vi "LVFunction_Imop_SlopesCompute_ModalCoef.vi"(0 "HasoSlopes IN":refnum<class "HasoSlopes.lvclass">, 5 "ComputePhaseSet":refnum<class "ComputePhaseSet.lvclass">, 7 "ModalCoef  IN":refnum<class "ModalCoef.lvclass">, 11 "error constant":errorcluster) -> (4 "HasoSlopes (dup)":refnum<class "HasoSlopes.lvclass">, 6 "ComputePhaseSet.lvclass (dup)":refnum<class "ComputePhaseSet.lvclass">, 8 "ModalCoef OUT":refnum<class "ModalCoef.lvclass">, 15 "error out":errorcluster)   [LabVIEW 2020]
doc: "Compute modal coefficients that represent the processed slopes of the input\nslopes data in a given basis of polynomials provided by ComputePhaseSet.\n\n<B>ComputePhaseSetIn</B> : ComputePhaseSet object.\n<B>ComputePhaseSetOut</B> : ComputePhaseSet object.\n<B>HasoData</B> : Slopes object.\n<B>ModalCoeffs</B> : ModalCoef object. Preferences are used as input, coefficients values are updated by the processing."
uses:
  HasoSlopes.lvclass
  ComputePhaseSet.lvclass
  ModalCoef.lvclass
  LVClass_ModalCoef Read ModalCoef.vi
  LVClass_ComputePhaseSet Read ComputePhaseSet.vi
  LVClass_HasoSlopes Read HasoSlopes _ property.vi
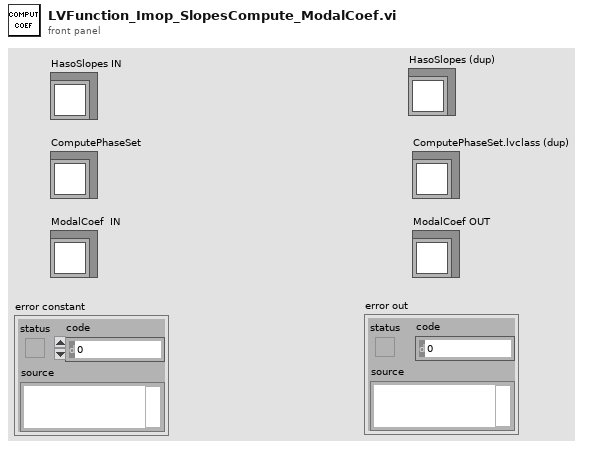
[diagram p1: front panel]
types:
  T1 = typedef "ClassID.ctl" = i64
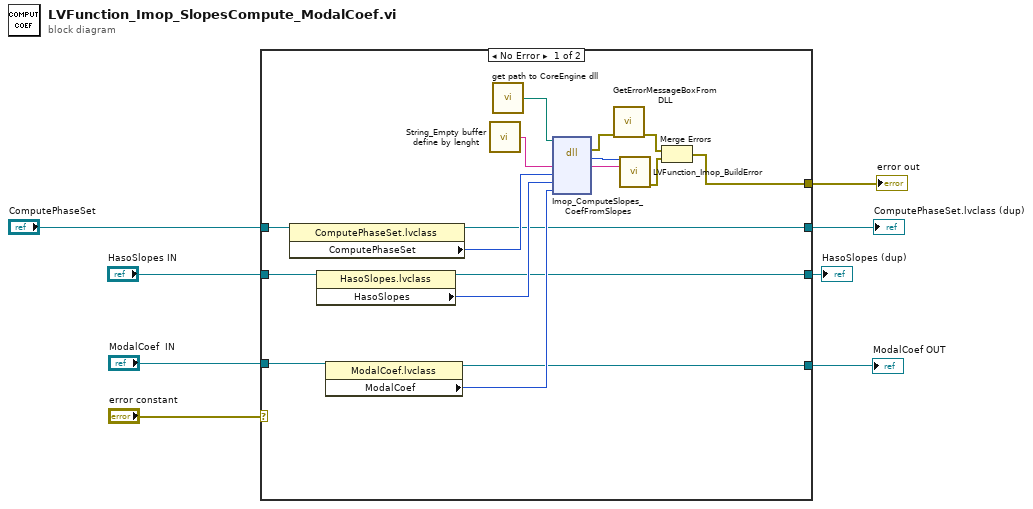
[diagram p0: block diagram]
diagram:
  n1 = case shown="No Error" "error constant" {
    selector: "error constant" -> [_ w29]
    tunnel: "HasoSlopes IN" -> [w20 w26]
    tunnel: "ComputePhaseSet" -> [w19 w28]
    tunnel: [w12 w29] -> w7
    tunnel: "ModalCoef  IN" -> [w16 w27]
    tunnel: [w11 w27] -> w3
    tunnel: [w10 w28] -> w2
    tunnel: [w9 w26] -> w1
    frame No Error {
      n2 = property class="ComputePhaseSet.lvclass"(reference=w19) -> (reference out=w10:refnum<class "ComputePhaseSet.lvclass">, "ComputePhaseSet"=w18:T1)  [unwired: 1 in, 1 out]
      n3 = property class="HasoSlopes.lvclass"(reference=w20) -> (reference out=w9:refnum<class "HasoSlopes.lvclass">, "HasoSlopes"=w17:T1)  [unwired: 1 in, 1 out]
      n4 = property class="ModalCoef.lvclass"(reference=w16) -> (reference out=w11:refnum<class "ModalCoef.lvclass">, "ModalCoef"=w15:T1)  [unwired: 1 in, 1 out]
      n5 = call "String_Empty buffer define by lenght.vi"() -> ("Empty buffer"=w23:string)  [unwired: 1 in]
      n6 = call "get path to CoreEngine dll.vi"() -> ("path to wavekit library"=w22:path)  [unwired: 14 in, 1 out]
      n7 = dll-call lib="D:/FLE/0.Code/CoreEngine4_Suite/LV2011_interface/DLLs/c_interface_vc100.dll" fn="Imop_ComputeSlopes_CoefFromSlopes"(path in=w22, "message"=w23, "ComputePhaseSet"=w18, "HasoSlopes"=w17, "ModalCoeffs"=w15) -> (error out=w21:errorcluster, "return type"=w25:i32, "message"=w24:string)  [unwired: 5 in, 1 out]
      n8 = call "GetErrorMessageBoxFromDLL.vi"("error IN"=w21) -> ("error OUT"=w14:errorcluster)  [unwired: 10 in]
      n9 = call "LVFunction_Imop_BuildError.vi"("code"=w25, "String to Prepend to source (\"\")"=w24) -> ("error out"=w13:errorcluster)  [unwired: 13 in]
      n10 = Merge Errors(w14, w13) -> (w12:errorcluster)
    }
    frame Error {
    }
  }
  "error out" <- w7
  "ModalCoef OUT" <- w3
  "ComputePhaseSet.lvclass (dup)" <- w2
  "HasoSlopes (dup)" <- w1
